vi "Init.vi"(4 "CS Active Low (T)":bool=TRUE, 5 "CS GPIO (None)":T1=-1, 7 "SPI #":T2=-1, 8 "error in (no error)":errorcluster, 10 "Session":refnum<class "Session.lvclass">) -> (0 "error out":errorcluster, 3 "SPI Connection":refnum<class "SPI Connection.lvclass">)   [LabVIEW 2024, in "CTI.lvlib" / "SPI Connection.lvclass"]
uses:
  SPI Connection.lvclass
  SPI Number.ctl
  GPIO Number.ctl
  Session/Session.lvclass
  SPI Connection.lvclass/SPI Connection.ctl
  CTI.lvlib
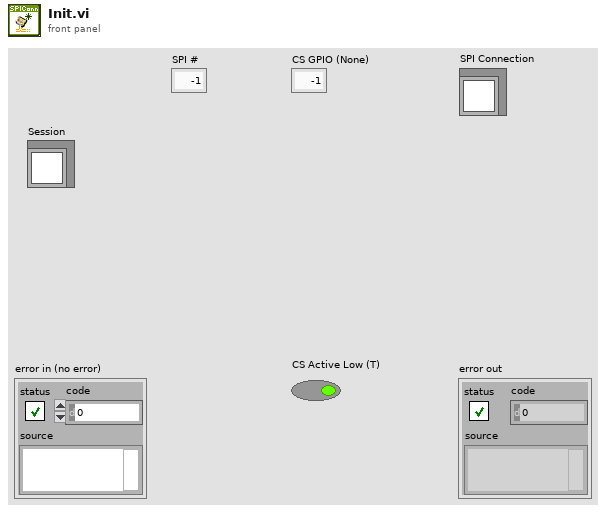
[diagram p1: front panel]
types:
  T1 = typedef "CTI.lvlib/GPIO Number.ctl" = i8
  T2 = typedef "CTI.lvlib/SPI Number.ctl" = i8
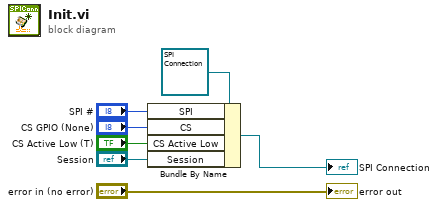
[diagram p0: block diagram]
diagram:
  n1 = Bundle By Name(cluster=refnum<class "SPI Connection.lvclass"> refnum ("SPI Device in"), "SPI"="SPI #", "CS"="CS GPIO (None)", "CS Active Low"="CS Active Low (T)", "Session"="Session") -> (→"SPI Connection":refnum<class "SPI Connection.lvclass">)
  "error out" <- "error in (no error)"
